vi "Count Two Phase Digital Encoder.vi"(4 "initial count (0)":i32, 5 "cycles to filter (0)":u16, 6 "reset (F)":bool, 7 "count encoding (X1)":T1, 10 "phase B FPGA digital input":refnum<k21>="Port0/DIO1", 11 "phase A FPGA digital input":refnum<k21>="Port0/DIO0") -> (2 "count change":i32, 3 "new count":i32)   [LabVIEW 2017, in "NI_Robotics_FPGA Utilities.lvlib"]
uses:
  <vilib>/robotics/Utilities/FPGA Utilities/NI_Robotics_FPGA Utilities.lvlib
  <vilib>/robotics/Utilities/NI_Robotics Utilities.lvlib
  <vilib>/robotics/Utilities/Encoder Count Encoding.ctl
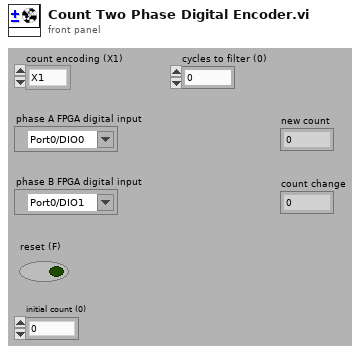
[diagram p1: front panel]
types:
  T1 = typedef "NI_Robotics Utilities.lvlib/Encoder Count Encoding.ctl" = enum16{"X1", "X2", "X4"}
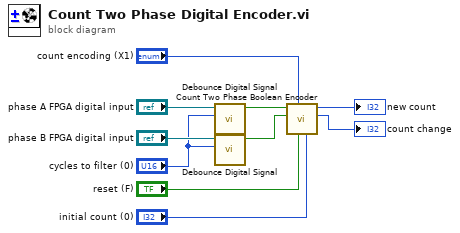
[diagram p0: block diagram]
diagram:
  n1 = call <vilib>:"Debounce Digital Signal.vi"("cycles to filter (0)"="cycles to filter (0)", "FPGA digital input"="phase A FPGA digital input") -> ("filtered output"=w5:bool)  [unwired: 9 in]
  n2 = call <vilib>:"Debounce Digital Signal.vi"("cycles to filter (0)"="cycles to filter (0)", "FPGA digital input"="phase B FPGA digital input") -> ("filtered output"=w3:bool)  [unwired: 9 in]
  n3 = call <vilib>:"Count Two Phase Boolean Encoder.vi"("initial count (0)"="initial count (0)", "reset (F)"="reset (F)", "count encoding (X1)"="count encoding (X1)", "phase B"=w3, "phase A"=w5) -> ("count change"=→"count change":i32, "new count"=→"new count":i32)  [unwired: 5 in]
